vi "find subscription nodes.vi"(8 "error in":errorcluster, 10 "Command":string, 11 "refnum in":T1) -> (0 "error out":errorcluster, 2 "Subscribers[]":string[](array[string]), 3 "refnum in":T1)   [LabVIEW 2023, in "Publisher Subscriber.lvlib"]
uses:
  <userlib>/_Publisher Subscriber/Publisher Subscriber.lvlib
  <userlib>/_Publisher Subscriber/Controls/node refnum.ctl
  <userlib>/_Publisher Subscriber/Controls/node dvr data.ctl
  <userlib>/_Publisher Subscriber/Controls/data cluster.ctl
  <userlib>/_Publisher Subscriber/Controls/subscription bank ref.ctl
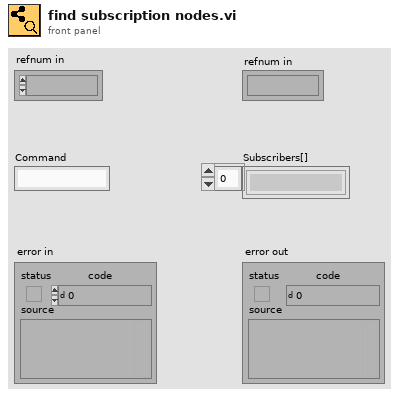
[diagram p1: front panel]
types:
  T1 = typedef "Publisher Subscriber.lvlib/node refnum.ctl" = refnum<vi>
  T2 = typedef "Publisher Subscriber.lvlib/node dvr data.ctl" = cluster{"queue ref":refnum<queue>, "Subscription Bank Ref":refnum<data-value>, "Command":string, "Data":variant, "Subscriptions []":set{string}, "Variables DVR Ref":refnum<data-value>}
  T3 = typedef "Publisher Subscriber.lvlib/subscription bank ref.ctl" = map{string, set{refnum<queue>}}
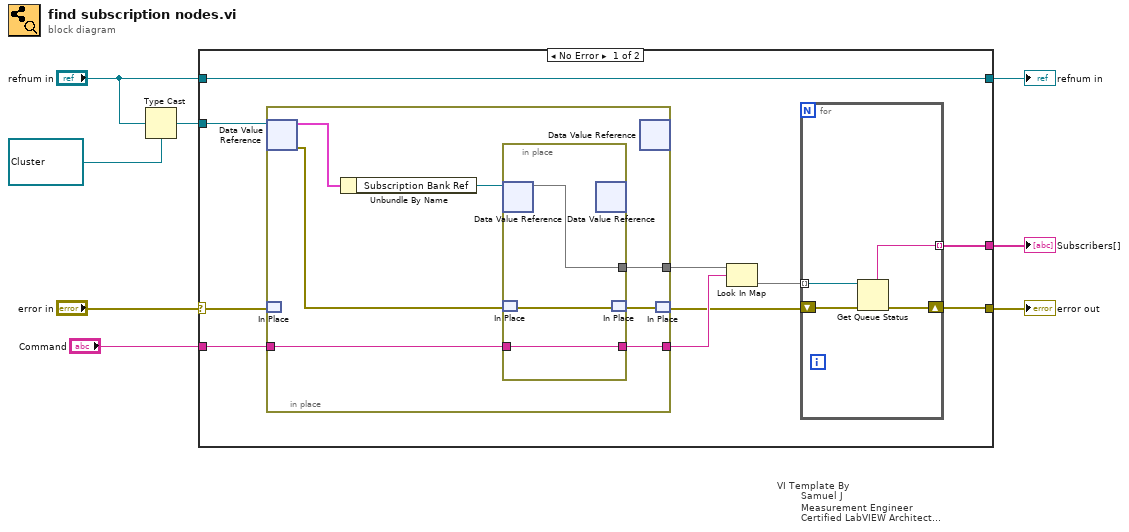
[diagram p0: block diagram]
diagram:
  n1 = Type Cast(type=refnum<data-value> refnum ("data value reference"), x="refnum in") -> (*(type *) &x=w6:refnum<data-value>)
  n2 = case "VI Template By\n        Samuel J\n        Measurement Engineer\n        Certified LabVIEW Architect\n        Vestas Technology R&D Chennai" shown="No Error" "error in" {
    selector: "error in" -> [w16 w34]
    tunnel: [w10 w34] -> w1
    tunnel: w6 -> [w17 _]
    tunnel: [w18 w33] -> w5
    tunnel: "refnum in" -> [w18 w33]
    tunnel: [w9 _] -> w3
    tunnel: "Command" -> [w15 _]
    frame No Error {
      n3 = in-place {
        in-place-border: [w21] -> w13
        in-place-border: w15 -> [w20]
        in-place-border: [w19] -> w12
        n4 = in-place-dvr #1(w17) -> (w25:T2, w23:errorcluster)
        n5 = in-place-match #2(w16) -> ()  [unwired: 1 out]
        n6 = Unbundle By Name(w25) -> ("Subscription Bank Ref"=w24:refnum<data-value>)
        n7 = in-place {
          in-place-border: [w27] -> w21
          in-place-border: w20 -> [w26]
          in-place-border: [w26] -> w19
          n8 = in-place-dvr #3(w24) -> (w27:T3)  [unwired: 1 out]
          n9 = in-place-match #4(w23) -> (w28:errorcluster)
          n10 = in-place-dvr #3() -> ()  [unwired: 1 in, 2 out]
          n11 = in-place-match #4(w28) -> (w22:errorcluster)
        }
        n12 = in-place-dvr #1() -> ()  [unwired: 1 in, 2 out]
        n13 = in-place-match #2(w22) -> (w11:errorcluster)
      }
      n14 = Look In Map(map=w13, key=w12) -> (value=w14:set{refnum<queue>})  [unwired: 1 in, 1 out]
      n15 = for {
        shift-right: [w32] -> w10
        shift-left: w11 -> [w31]
        tunnel: w14 -> [w30] mode=indexing
        tunnel: [w29] -> w9 mode=indexing
        n16 = Get Queue Status(queue=w30, error in (no error)=w31) -> (queue name=w29:string, error out=w32:errorcluster)  [unwired: 1 in, 6 out]
      }
    }
    frame Error {
    }
  }
  "error out" <- w1
  "refnum in" <- w5
  "Subscribers[]" <- w3
